vi "SubSystems.vi"(8 "error in":errorcluster) -> ()   [LabVIEW 2017]
doc: "This VI calls the various robot subsystems that will then run in parallel. New subSystems will automatlically script code to make the call."
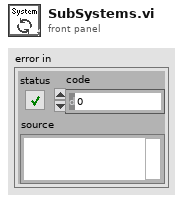
[diagram p1: front panel]
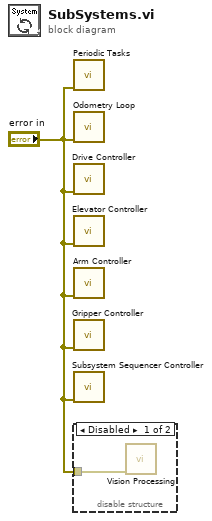
[diagram p0: block diagram]
diagram:
  n1 = call "Periodic Tasks.vi"("error in"="error in") -> ()  [unwired: 1 in, 10 out]
  n2 = call "Odometry Loop.vi"("error in (no error)"="error in") -> ()  [unwired: 9 in]
  n3 = call "Drive Controller.vi"("error in"="error in") -> ()  [unwired: 11 in]
  n4 = call "Elevator Controller.vi"("error in"="error in") -> ()  [unwired: 11 in]
  n5 = call "Arm Controller.vi"("error in"="error in") -> ()  [unwired: 11 in]
  n6 = call "Gripper Controller.vi"("error in"="error in") -> ()  [unwired: 11 in]
  n7 = call "Subsystem Sequencer Controller.vi"("error in"="error in") -> ()  [unwired: 11 in]
  n8 = disable-structure shown="Disabled" {
    disable-tunnel: "error in" -> [w2 _]
    frame Disabled {
      n9 = call "Vision Processing.vi"("error in (no error)"=w2) -> ()  [unwired: 7 in]
    }
    frame Enabled {
    }
  }
